vi "main_write_summary.vi"(10 "Runtime String":refnum<vi>) -> ()   [LabVIEW 2019]
uses:
  lib/libSimulationControl/libSimulationControl.lvlib
panel:
  # "*******************************************************************\nBiogas Plant Control\n\nAuthor: Paul Zügel\nGCSC-Frankfurt am Main 2020\n\n*******************************************************************"
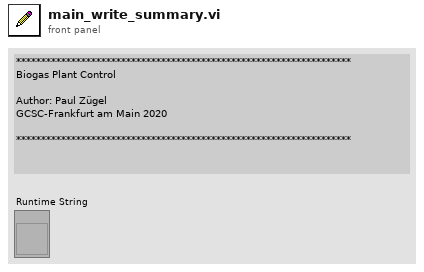
[diagram p1: front panel]
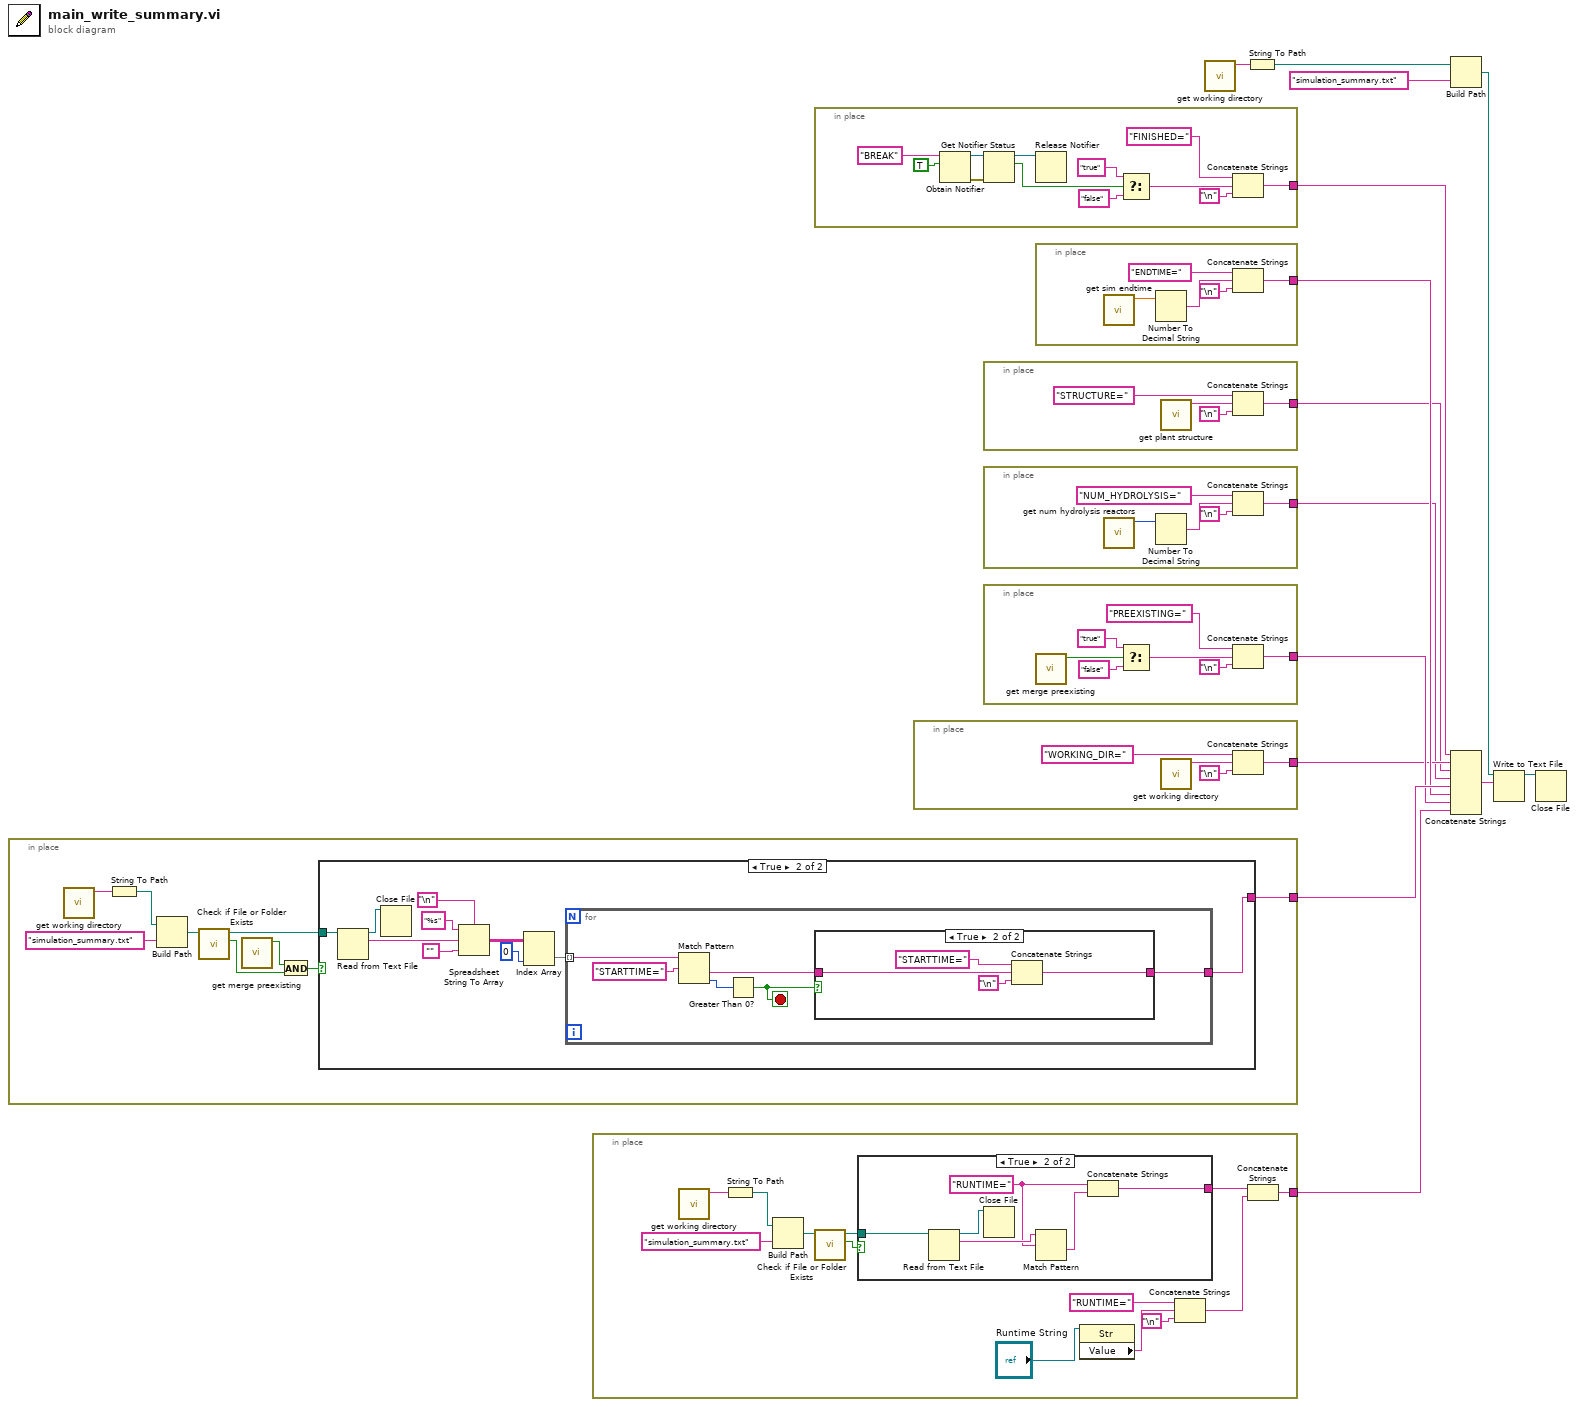
[diagram p0: block diagram]
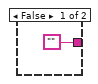
[diagram p2: hidden frame]
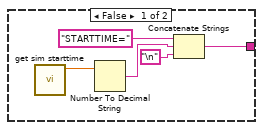
[diagram p3: hidden frame]
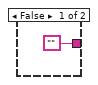
[diagram p4: hidden frame]
diagram:
  n1 = in-place {
    in-place-border: [w23] -> w10
    n2 = call "get working directory.vi"() -> ("function return"=w19:string)  [unwired: 10 in, 1 out]
    n3 = String To Path(string=w19) -> (path=w18:path)
    n4 = Build Path(base path=w18, name or relative path="simulation_summary.txt") -> (appended path=w20:path)
    n5 = call <vilib>:"Check if File or Folder Exists.vi"("path"=w20) -> ("file or folder exists?"=w22:bool, "dup path"=w15:path)  [unwired: 8 in, 1 out]
    n6 = call "get merge preexisting.vi"() -> ("function return"=w21:bool)  [unwired: 10 in, 1 out]
    n7 = And(x=w21, y=w22) -> (x .and. y?=w16:bool)
    n8 = case shown="True" w16 {
      tunnel: [w24 w30] -> w23
      tunnel: w15 -> [_ w38]
      frame False {
        n9 = call "get sim starttime.vi"() -> ("sim_starttime"=w26:dbl)  [unwired: 10 in, 1 out]
        n10 = Number To Decimal String(number=w26) -> (decimal integer string=w25:string)  [unwired: 1 in]
        n11 = Concatenate Strings("STARTTIME=" ("text"), w25, "\n") -> (w24:string)
      }
      frame True {
        n12 = Read from Text File(file (use dialog)=w38) -> (refnum out=w29:refnum<file>, text=w31:string)  [unwired: 3 in, 2 out]
        n13 = Close File(refnum=w29) -> ()  [unwired: 1 in, 2 out]
        n14 = Spreadsheet String To Array(delimiter (Tab)="\n", format string="%s", spreadsheet string=w31, array type (2D Dbl)="") -> (array=w36:string[][])
        n15 = Index Array(array=w36, index (col)=0 ("disabled index (col)")) -> (element=w37:string[])  [unwired: 1 in]
        n16 = for {
          tunnel: w37 -> [w44] mode=indexing
          tunnel: [w39] -> w30
          stop <- w40 stop-if-true
          n17 = Match Pattern(string=w44, regular expression="STARTTIME=") -> (after substring=w42:string, offset past match=w43:i32)  [unwired: 1 in, 2 out]
          n18 = Greater Than 0?(x=w43) -> (x > 0?=w40:bool)
          n19 = case shown="True" w40 {
            tunnel: w42 -> [_ w47]
            tunnel: ["" w46] -> w39
            frame False {
            }
            frame True {
              n20 = Concatenate Strings("STARTTIME=" ("regular expression"), w47, "\n") -> (w46:string)
            }
          }
        }
      }
    }
  }
  n21 = in-place {
    in-place-border: [w50] -> w6
    n22 = call "get working directory.vi"() -> ("function return"=w56:string)  [unwired: 10 in, 1 out]
    n23 = String To Path(string=w56) -> (path=w57:path)
    n24 = Build Path(base path=w57, name or relative path="simulation_summary.txt") -> (appended path=w55:path)
    n25 = call <vilib>:"Check if File or Folder Exists.vi"("path"=w55) -> ("file or folder exists?"=w54:bool, "dup path"=w53:path)  [unwired: 8 in, 1 out]
    n26 = case shown="True" w54 {
      tunnel: w53 -> [_ w69]
      tunnel: ["" w65] -> w52
      frame False {
      }
      frame True {
        w66 = "RUNTIME=" ("regular expression")
        n27 = Read from Text File(file (use dialog)=w69) -> (refnum out=w64:refnum<file>, text=w68:string)  [unwired: 3 in, 2 out]
        n28 = Close File(refnum=w64) -> ()  [unwired: 1 in, 2 out]
        n29 = Match Pattern(string=w68, regular expression=w66) -> (after substring=w67:string)  [unwired: 1 in, 3 out]
        n30 = Concatenate Strings(w66, w67) -> (w65:string)
      }
    }
    n31 = property class="Str"(reference="Runtime String") -> ("Value"=w59:string)  [unwired: 1 in, 2 out]
    n32 = Concatenate Strings("RUNTIME=" ("text"), w59, "\n") -> (w51:string)
    n33 = Concatenate Strings(w52, w51) -> (w50:string)
  }
  n34 = in-place {
    in-place-border: [w71] -> w5
    n35 = Obtain Notifier(name (unnamed)="BREAK", notification data type=TRUE) -> (notifier out=w79:refnum<notifier>, error out=w78:errorcluster)  [unwired: 2 in, 1 out]
    n36 = Get Notifier Status(notifier=w79, error in (no error)=w78) -> (notifier out=w70:refnum<notifier>, current notification=w75:bool)  [unwired: 3 out]
    n37 = Release Notifier(notifier=w70) -> ()  [unwired: 2 in, 3 out]
    n38 = Select(t="true", s=w75, f="false") -> (s? t:f=w72:string)
    n39 = Concatenate Strings("FINISHED=" ("text"), w72, "\n") -> (w71:string)
  }
  n40 = in-place {
    in-place-border: [w82] -> w4
    n41 = call "get working directory.vi"() -> ("function return"=w83:string)  [unwired: 10 in, 1 out]
    n42 = Concatenate Strings("WORKING_DIR=" ("text"), w83, "\n") -> (w82:string)
  }
  n43 = in-place {
    in-place-border: [w86] -> w3
    n44 = call "get plant structure.vi"() -> ("function return"=w88:string)  [unwired: 10 in, 1 out]
    n45 = Concatenate Strings("STRUCTURE=" ("text"), w88, "\n") -> (w86:string)
  }
  n46 = in-place {
    in-place-border: [w92] -> w2
    n47 = call "get num hydrolysis reactors.vi"() -> ("function return"=w91:i32)  [unwired: 10 in, 1 out]
    n48 = Number To Decimal String(number=w91) -> (decimal integer string=w90:string)  [unwired: 1 in]
    n49 = Concatenate Strings("NUM_HYDROLYSIS=" ("text"), w90, "\n") -> (w92:string)
  }
  n50 = in-place {
    in-place-border: [w95] -> w8
    n51 = call "get merge preexisting.vi"() -> ("function return"=w99:bool)  [unwired: 10 in, 1 out]
    n52 = Select(t="true", s=w99, f="false") -> (s? t:f=w96:string)
    n53 = Concatenate Strings("PREEXISTING=" ("text"), w96, "\n") -> (w95:string)
  }
  n54 = in-place {
    in-place-border: [w102] -> w9
    n55 = call "get sim endtime.vi"() -> ("function return"=w103:dbl)  [unwired: 10 in, 1 out]
    n56 = Number To Decimal String(number=w103) -> (decimal integer string=w104:string)  [unwired: 1 in]
    n57 = Concatenate Strings("ENDTIME=" ("text"), w104, "\n") -> (w102:string)
  }
  n58 = call "get working directory.vi"() -> ("function return"=w11:string)  [unwired: 10 in, 1 out]
  n59 = String To Path(string=w11) -> (path=w12:path)
  n60 = Build Path(base path=w12, name or relative path="simulation_summary.txt") -> (appended path=w14:path)
  n61 = Concatenate Strings(w5, w4, w3, w2, w10, w9, w8, w6) -> (w7:string)
  n62 = Write to Text File(file (use dialog)=w14, text=w7) -> (refnum out=w1:refnum<file>)  [unwired: 2 in, 2 out]
  n63 = Close File(refnum=w1) -> ()  [unwired: 1 in, 2 out]
